vi "ClearDMA_5782.vi"(8 "error in":errorcluster, 11 "scope in":T1) -> (0 "error out":errorcluster, 3 "scope out":T1)   [LabVIEW 2013]
uses:
  controls/scope_params_5782.ctl
  Utilities/Ticker/Ticker.lvclass
  Communication/Driver/RemoteConnection/RemoteConnection.lvclass
  Scope/controls/ScopeMode.ctl
  Config/FPGAref_5782.ctl
  FPGA/DataMode.ctl
  controls/5782_trigger_type.ctl
  <vilib>/rvi/interface/common/niFpgaWaitOnOcc.vi
  <vilib>/Utility/error.llb/Error Cluster From Error Code.vi
  <vilib>/rvi/errors/niLvFpgaAdjustHostInterfaceError.vi
  <vilib>/rvi/interface/nirviMethod/nirviMethod.xnode
  <vilib>/FPGAPlugInAG/Dynamic/niLvFpga_ReadFifo_Dynamic.vi
  <vilib>/rvi/errors/niLvFpgaMergeErrorWithErrorCode.vi
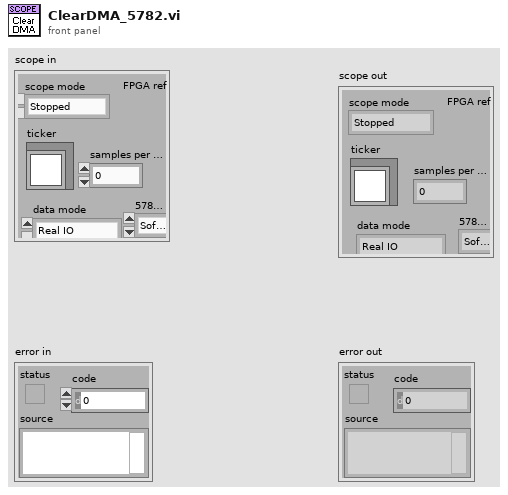
[diagram p1: front panel]
types:
  T1 = typedef "scope_params_5782.ctl" = cluster{"scope mode":T2, "ticker":refnum<class "Ticker.lvclass">, "samples per record":i32, "FPGA ref":T3, "data mode":T4, "5782 Trigger":T5, "Chart length":i32, "RemoteConnection":refnum<class "RemoteConnection.lvclass">}
  T2 = typedef "ScopeMode.ctl" = enum16{"Stopped", "Single", "Running", "Continuous"}
  T3 = typedef "FPGAref_5782.ctl" = refnum<k20>
  T4 = typedef "DataMode.ctl" = enum16{"Real IO", "Simulated"}
  T5 = typedef "5782_trigger_type.ctl" = enum16{"Software", "Trigger input"}
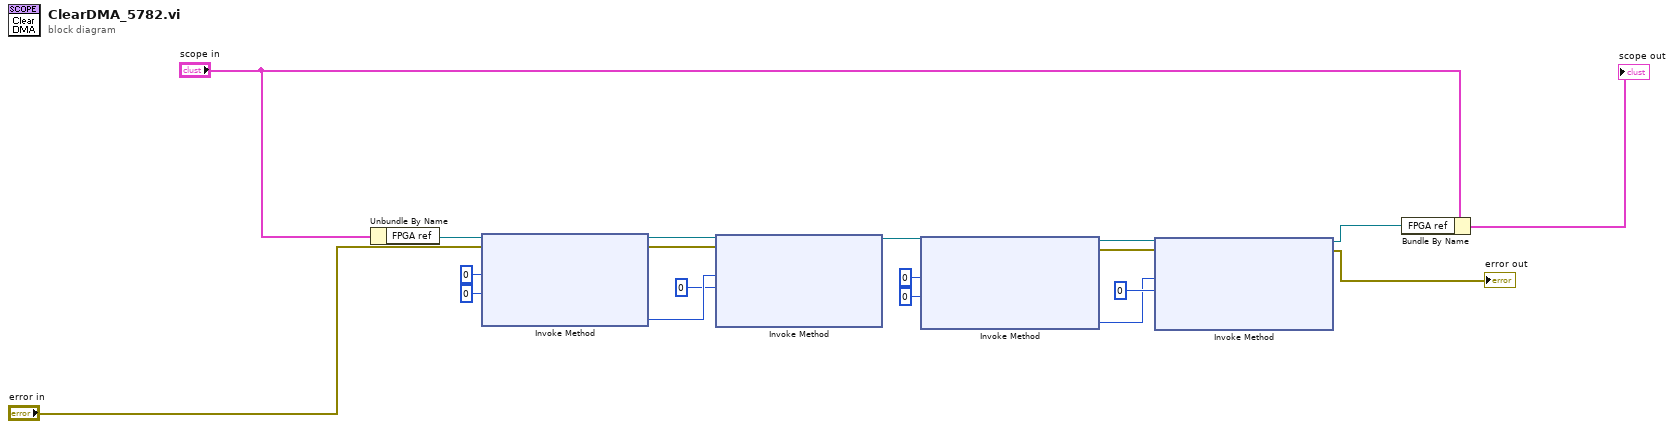
[diagram p0: block diagram]
diagram:
  n1 = Unbundle By Name("scope in") -> ("FPGA ref"=w11:T3)
  n2 = xnode "Invoke Method"("FPGA VI Reference In"=w11, "error in"="error in", "Number of Elements"=u32 0, "Timeout (ms)"=0) -> ("FPGA VI Reference Out"=w13:T3, "error out"=w12:errorcluster, "Elements Remaining"=w15:u32)  [unwired: 1 out]
  n3 = xnode "Invoke Method"("FPGA VI Reference In"=w13, "error in"=w12, "Number of Elements"=w15, "Timeout (ms)"=0) -> ("FPGA VI Reference Out"=w3:T3)  [unwired: 3 out]
  n4 = xnode "Invoke Method"("FPGA VI Reference In"=w3, "Number of Elements"=u32 0, "Timeout (ms)"=0) -> ("FPGA VI Reference Out"=w8:T3, "error out"=w9:errorcluster, "Elements Remaining"=w6:u32)  [unwired: 1 in, 1 out]
  n5 = xnode "Invoke Method"("FPGA VI Reference In"=w8, "error in"=w9, "Number of Elements"=w6, "Timeout (ms)"=0) -> ("FPGA VI Reference Out"=w2:T3, "error out"=→"error out":errorcluster)  [unwired: 2 out]
  n6 = Bundle By Name(cluster="scope in", "FPGA ref"=w2) -> (→"scope out":T1)
